vi "Math-Robust Loess.vi"(6 "NumIter":i32=5, 8 "Quadratic?":bool, 9 "Span":i32, 10 "Nonrobust Smoothed":dbl[](array[numeric]), 11 "Array":dbl[](array[numeric])) -> (3 "Robust Smoothed":dbl[](array[numeric]))   [LabVIEW 2020]
uses:
  LinSpace (x0-dx-npts).vi
  <vilib>/Analysis/7linalg.llb/Solve Linear Equations (single right hand).vi
  <vilib>/Analysis/baseanly.llb/Solve Linear Equations By Cholesky.vi
  <vilib>/Analysis/baseanly.llb/Real Matrix to Compact Array.vi
  <vilib>/Analysis/baseanly.llb/Real Compact Tri-Matrix Linear Eqs.vi
  Array Manipulation VIs/Irregular Array Subset (DBL).vi
  Array Manipulation VIs/Array-Dimensions (2D).vi
  <vilib>/Analysis/7linalg.llb/Solve Linear Eqs (General).vi
  <vilib>/Analysis/7linalg.llb/Solve Linear Eqs (Gen, single right hand).vi
  <vilib>/Analysis/NI_AALPro.lvlib
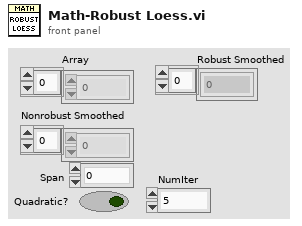
[diagram p1: front panel]
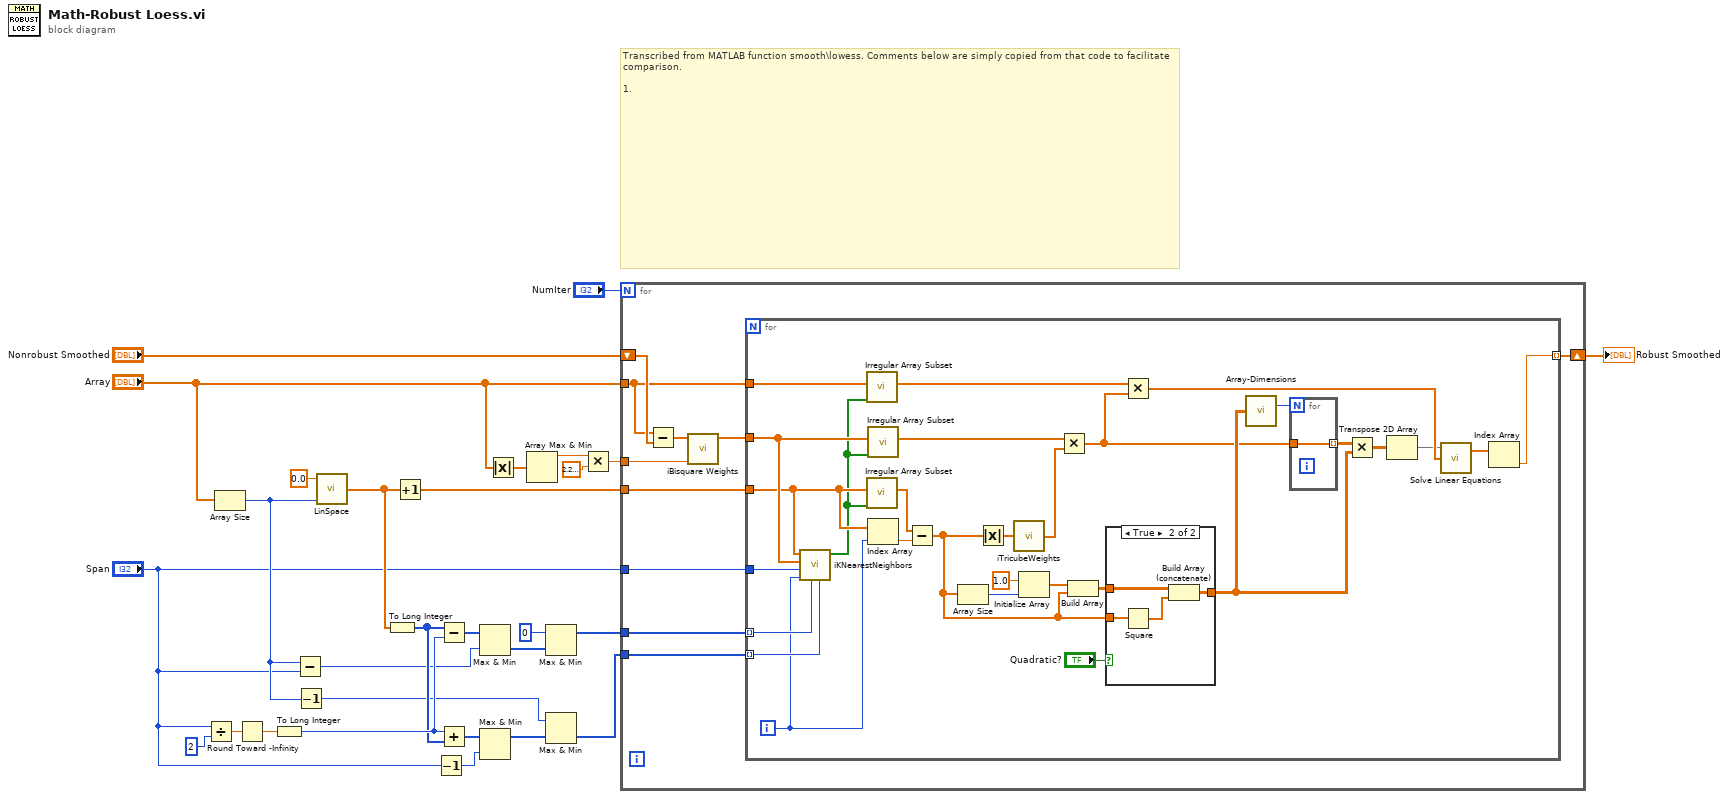
[diagram p0: block diagram]
diagram:
  # "Transcribed from MATLAB function smooth\\lowess. Comments below are simply copied from that code to facilitate comparison.\n\n1."
  n1 = Divide(x="Span", y=2) -> (x/y=w27:dbl)
  n2 = Array Size(array="Array") -> (size(s)=w15:i32)
  n3 = Round Toward -Infinity(1:w27) -> (0:w26:dbl)
  n4 = To Long Integer(number=w26) -> (32bit integer=w24:i32)
  n5 = Subtract(x=w15, y="Span") -> (x-y=w21:i32)
  n6 = Decrement(x=w15) -> (x-1=w14:i32)
  n7 = call-poly "LinSpace.vi"("npts"=w15, "x0"=0.0) -> ("Array"=w13:dbl[])  [unwired: 2 in, 1 out]
  n8 = To Long Integer(number=w13) -> (32bit integer=w23:i32[])
  n9 = Increment(x=w13) -> (x+1=w4:dbl[])
  n10 = Decrement(x="Span") -> (x-1=w19:i32)
  n11 = Subtract(x=w23, y=w24) -> (x-y=w22:i32[])
  n12 = Add(x=w24, y=w23) -> (x+y=w20:i32[])
  n13 = Max & Min(x=w22, y=w21) -> (min(x,y)=w18:i32[])  [unwired: 1 out]
  n14 = Max & Min(x=w20, y=w19) -> (max(x,y)=w16:i32[])  [unwired: 1 out]
  n15 = Absolute Value(x="Array") -> (abs(x)=w8:dbl[])
  n16 = Array Max & Min(array=w8) -> (max value=w7:dbl)  [unwired: 3 out]
  n17 = Max & Min(x=0, y=w18) -> (max(x,y)=w2:i32[])  [unwired: 1 out]
  n18 = Max & Min(x=w14, y=w16) -> (min(x,y)=w1:i32[])  [unwired: 1 out]
  n19 = Multiply(x=w7, y=2.220446049250313e-16) -> (x*y=w5:dbl)
  n20 = for {
    N: "NumIter" -> [_]
    tunnel: "Array" -> [w31]
    shift-right: [w35] -> w10
    shift-left: "Nonrobust Smoothed" -> [w36]
    tunnel: w5 -> [w37]
    tunnel: w2 -> [w34]
    tunnel: w1 -> [w33]
    tunnel: w4 -> [w30]
    tunnel: "Span" -> [w29]
    n21 = Subtract(x=w31, y=w36) -> (x-y=w38:dbl[])
    n22 = call "iBisquare Weights.vi"("my eps"=w37, "Array"=w38) -> ("Weights"=w32:dbl[])  [unwired: 9 in]
    n23 = for {
      tunnel: [w47] -> w35 mode=indexing
      tunnel: w34 -> [w67] mode=indexing
      tunnel: w33 -> [w66] mode=indexing
      tunnel: w32 -> [w46]
      tunnel: w31 -> [w45]
      tunnel: w30 -> [w44]
      tunnel: w29 -> [w65]
      i -> [w64]
      n24 = call "iKNearestNeighbors.vi"("Nominal End"=w66, "Nominal Start"=w67, "Index"=w64, "Span"=w65, "Weights"=w46, "X"=w44) -> ("Nearest Neighbors Mask"=w43:bool[])  [unwired: 5 in]
      n25 = call-poly "Irregular Array Subset.vi"("Mask"=w43, "Array"=w45) -> ("Array Subset"=w52:dbl[])  [unwired: 8 in, 1 out]
      n26 = call-poly "Irregular Array Subset.vi"("Mask"=w43, "Array"=w44) -> ("Array Subset"=w56:dbl[])  [unwired: 8 in, 1 out]
      n27 = call-poly "Irregular Array Subset.vi"("Mask"=w43, "Array"=w46) -> ("Array Subset"=w42:dbl[])  [unwired: 8 in, 1 out]
      n28 = Index Array(array=w44, index=w64) -> (element=w63:dbl)
      n29 = Subtract(x=w56, y=w63) -> (x-y=w40:dbl[])
      n30 = Array Size(array=w40) -> (size(s)=w61:i32)
      n31 = Absolute Value(x=w40) -> (abs(x)=w62:dbl[])
      n32 = call "iTricubeWeights.vi"("Array"=w62) -> ("Weights"=w51:dbl[])
      n33 = Initialize Array(1.0 ("element"), w61) -> (w59:dbl[])
      n34 = Multiply(x=w42, y=w51) -> (x*y=w41:dbl[])
      n35 = Build Array(w59, w40) -> (w57:dbl[][])
      n36 = case shown="True" "Quadratic?" {
        tunnel: w57 -> [w69 w73]
        tunnel: w40 -> [_ w72]
        tunnel: [w69 w70] -> w53
        frame False {
        }
        frame True {
          n37 = Square(x=w72) -> (x^2=w71:dbl[])
          n38 = Build Array (concatenate)(w73, w71) -> (w70:dbl[][])
        }
      }
      n39 = Multiply(x=w52, y=w41) -> (x*y=w50:dbl[])
      n40 = call-poly "Array-Dimensions.vi"("2D Array"=w53) -> ("# rows"=w55:i32)  [unwired: 13 in, 1 out]
      n41 = for {
        N: w55 -> [_]
        tunnel: w41 -> [w68]
        tunnel: [w68] -> w54 mode=indexing
      }
      n42 = Multiply(x=w54, y=w53) -> (x*y=w49:dbl[][])
      n43 = Transpose 2D Array(2D array=w49) -> (transposed array=w39:dbl[][])
      n44 = call-poly <vilib>:"Solve Linear Equations.vi"("Known Vector"=w50, "Input Matrix"=w39) -> ("Solution Vector"=w48:dbl[])  [unwired: 1 in, 1 out]
      n45 = Index Array(array=w48) -> (element=w47:dbl)  [unwired: 1 in]
    }
  }
  "Robust Smoothed" <- w10
